vi "Evenly Divisible Check.vi"(1 "y":i32, 2 "x":i32) -> (0 "Evenly Divisible?":bool)   [LabVIEW 2018]
uses:
  <vilib>/rvi/Emulation/niFpgaGetClockAttributes.vi
  <vilib>/rvi/Emulation/niFpgaSctlEmulationGetInTimedLoop.vi
  <vilib>/rvi/Emulation/niFpgaEmulationReportErrorSimple.vi
  <vilib>/rvi/Emulation/niFpgaCriticalErrorInLSC.vi
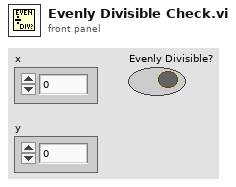
[diagram p1: front panel]
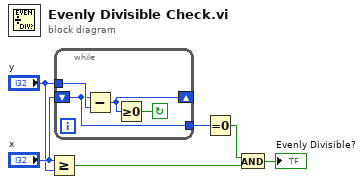
[diagram p0: block diagram]
diagram:
  n1 = Greater Or Equal?(x="x", y="y") -> (x >= y?=w3:bool)
  n2 = while {
    shift-right: [w8] -> _
    shift-left: "x" -> [w7]
    tunnel: "y" -> [w10]
    tunnel: [w7] -> w6
    stop <- w9 continue-if-true
    n3 = Subtract(x=w7, y=w10) -> (x-y=w8:i32)
    n4 = Greater Or Equal To 0?(x=w8) -> (x >= 0?=w9:bool)
  }
  n5 = Equal To 0?(x=w6) -> (x = 0?=w2:bool)
  n6 = And(x=w2, y=w3) -> (x .and. y?=→"Evenly Divisible?":bool)
